vi "Commas Needed.vi"(11 "Comma needed":bool) -> (3 "Comma Needed For Insert":T1)   [LabVIEW 2020, in "JSONtext.lvlib"]
uses:
  <vilib>/JDP Science/JSONtext/JSONtext.lvlib
  <vilib>/JDP Science/JSONtext/support/Comma Needed for Insert.ctl
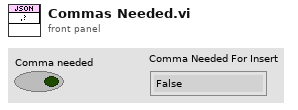
[diagram p1: front panel]
types:
  T1 = typedef "JSONtext.lvlib/Comma Needed for Insert.ctl" = enum8{"False", "True", "Following"}
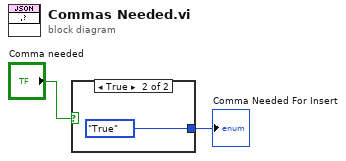
[diagram p0: block diagram]
diagram:
  n1 = case shown="True" "Comma needed" {
    tunnel: [_ Comma_Needed_for_Insert."True" ("Comma Needed For Insert")] -> w1
    frame False {
    }
    frame True {
    }
  }
  "Comma Needed For Insert" <- w1
